vi "elab pictures 3d.vi"(8 "error in":errorcluster, 11 "path file in":path) -> (0 "error out":errorcluster)   [LabVIEW 2023]
uses:
  listbox/Selection Global Method.ctl
  <vilib>/Utility/file.llb/Read Delimited Spreadsheet (I64).vi
  queue/Front Panel Message Queue.lvlib
panel:
  in  "Z Slice":i16
  out "all rows 2":i32[][][](array[numeric])
  out "all rows":i32[][][](array[numeric])
  in  "List Selected":T1(array[cluster])
  out "List Selected v":string[](array[string])
  out "List File":i32(listbox)
  in  "load":bool
  in  "Stop":bool
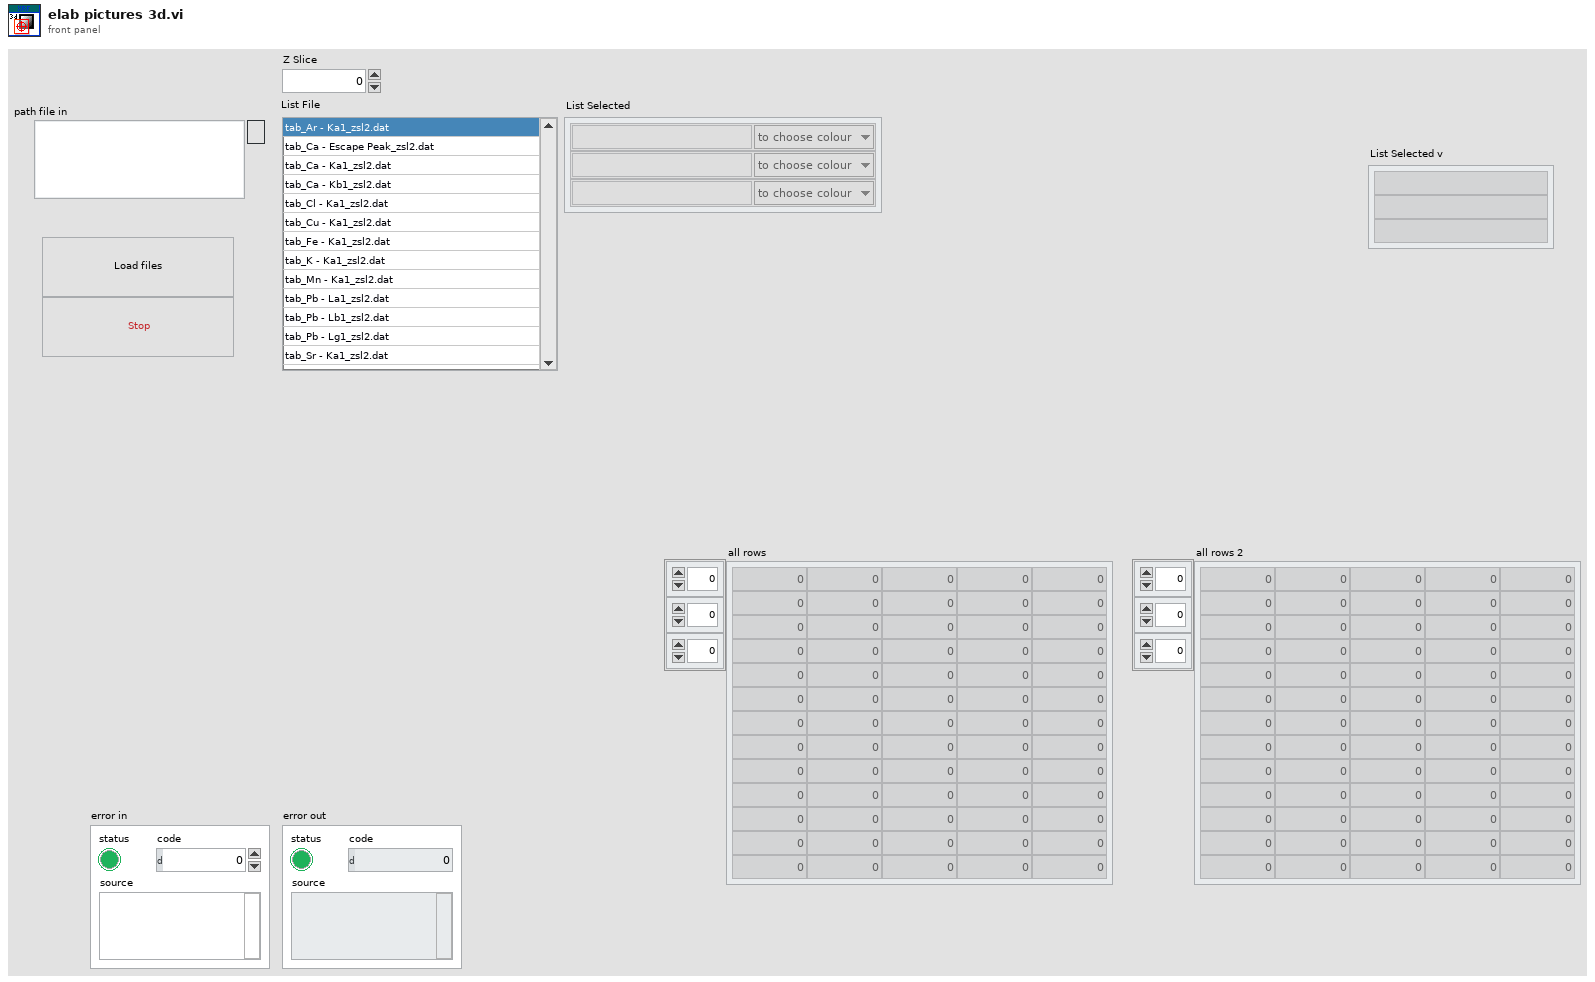
[diagram p1: front panel]
types:
  T1 = cluster{"Table":string, "color":enum16{"to choose colour", "red", "green", "blue"}}[]
  T2 = typedef "Front Panel Message Queue.lvlib/2d3d Message Queues.ctl" = cluster{"Main":refnum<queue>, "2d":refnum<queue>, "3d":refnum<queue>}
  T3 = typedef "Selection Global Method.ctl" = enum16{"Read Selection", "Force Selection", "Mouse Down Event", "Select All", "Select None", "Invert Selection", "Read Selection and Tags"}
  T4 = cluster{"Red name":string, "Green name":string, "Blu name":string}
  T5 = cluster{"Table":string, "color":enum16{"to choose colour", "red", "green", "blue"}}
  T6 = enum16{"to choose colour", "red", "green", "blue"}
  T7 = typedef "LVPoint32TypeDef.ctl" = cluster{"Horizontal":i32, "Vertical":i32}
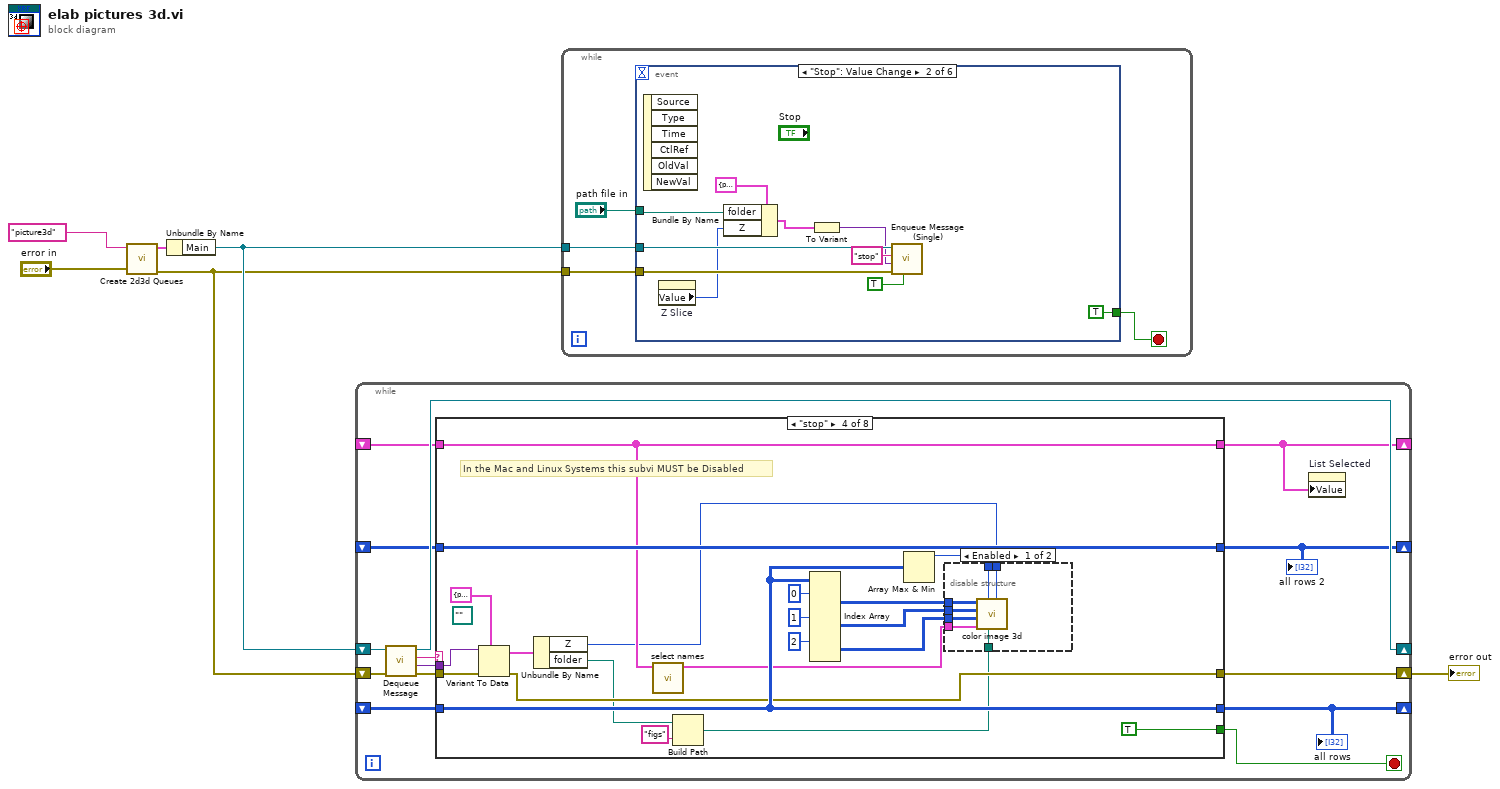
[diagram p0: block diagram]
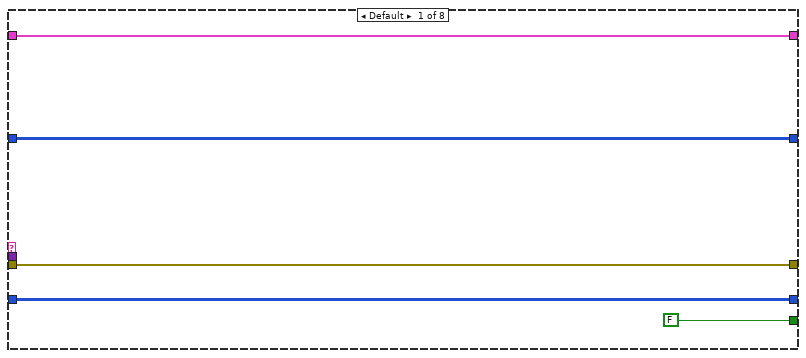
[diagram p2: hidden frame]
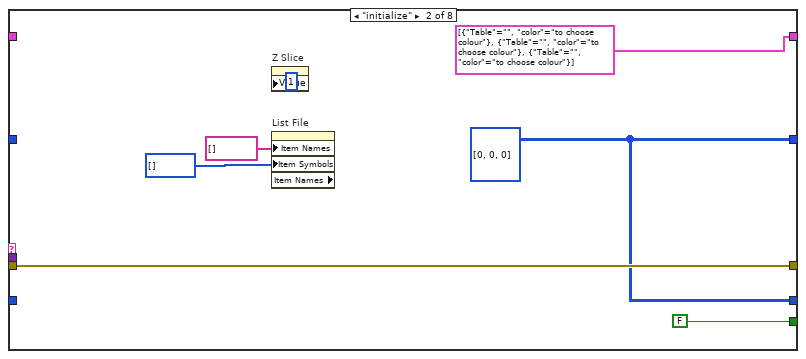
[diagram p3: hidden frame]
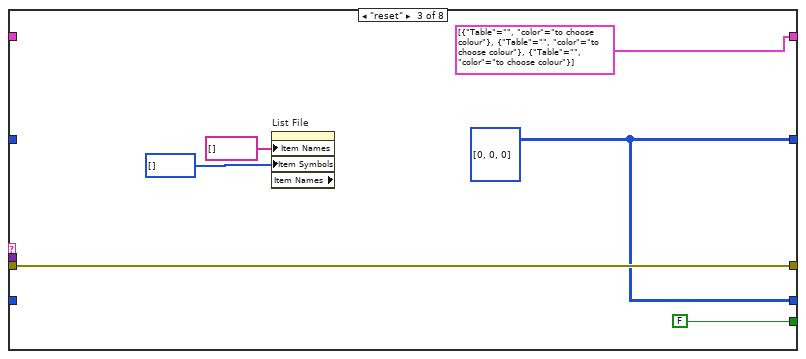
[diagram p4: hidden frame]
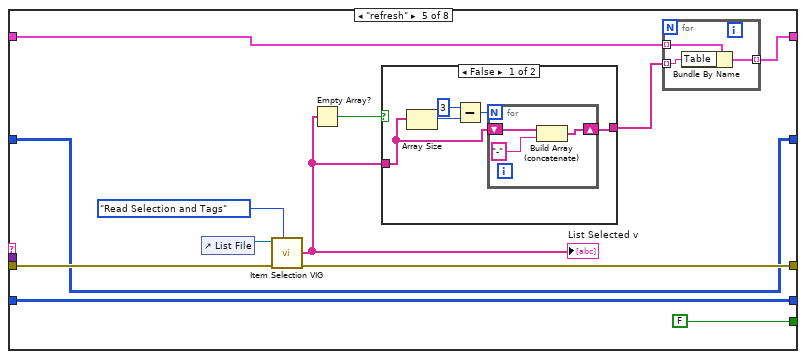
[diagram p6: hidden frame]
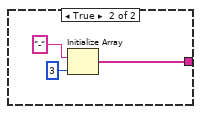
[diagram p7: hidden frame]
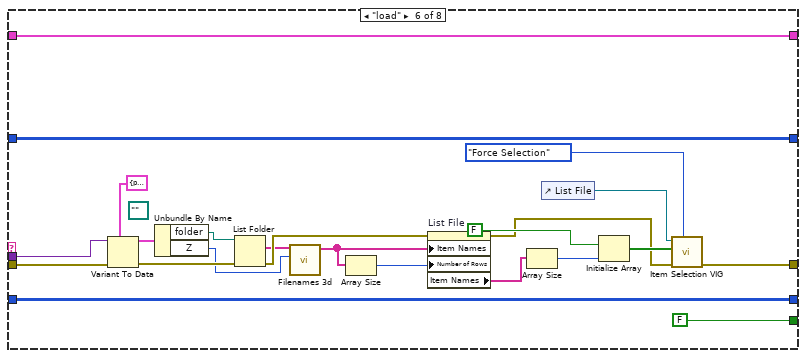
[diagram p8: hidden frame]
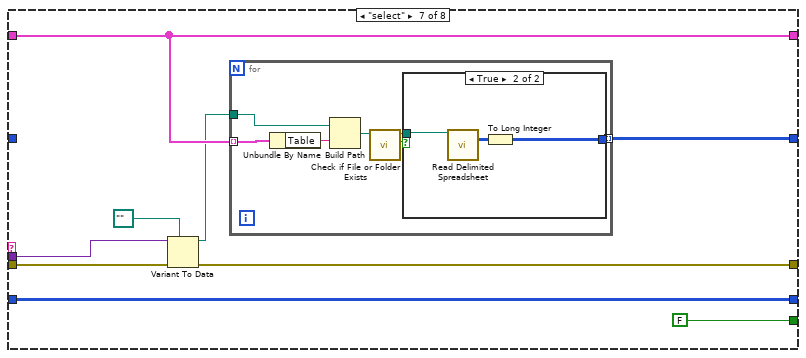
[diagram p9: hidden frame]
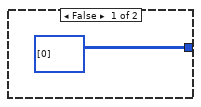
[diagram p10: hidden frame]
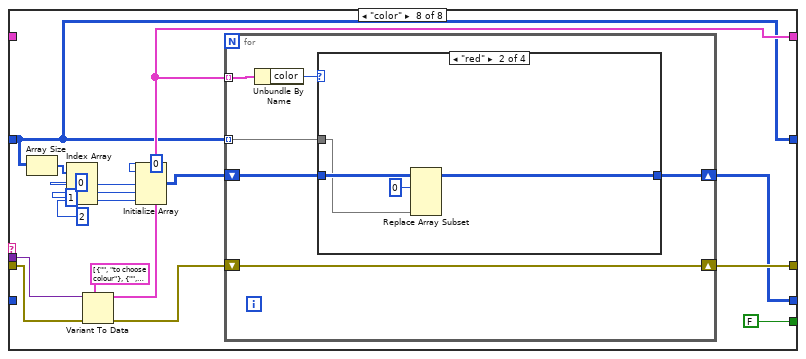
[diagram p11: hidden frame]
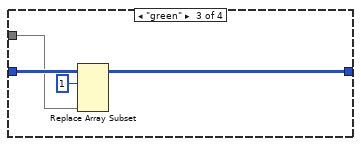
[diagram p13: hidden frame]
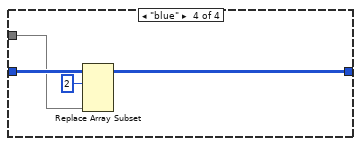
[diagram p14: hidden frame]
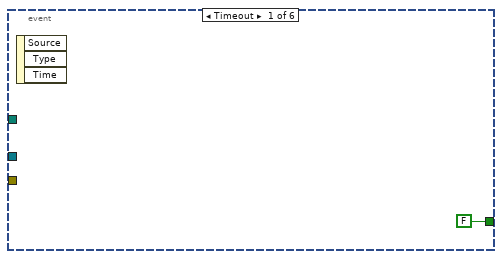
[diagram p15: hidden frame]
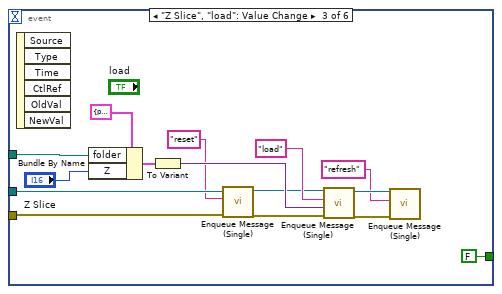
[diagram p16: hidden frame]
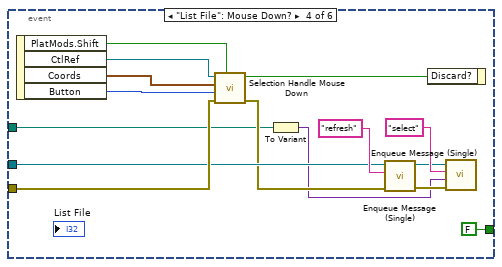
[diagram p17: hidden frame]
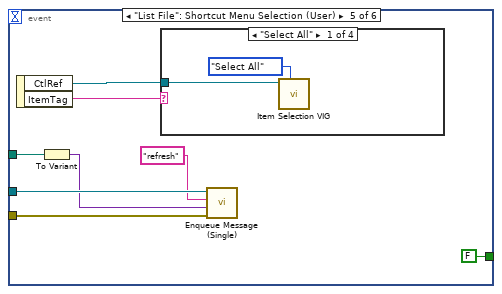
[diagram p18: hidden frame]
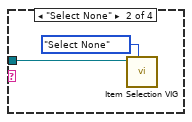
[diagram p19: hidden frame]
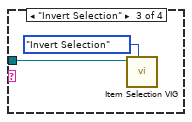
[diagram p20: hidden frame]
diagram:
  n1 = call "Create 2d3d Queues.vi"("error in (no error)"="error in", "name"="picture3d") -> ("error out"=w2:errorcluster, "Message Queues"=w4:T2)  [unwired: 8 in]
  n2 = Unbundle By Name(w4) -> ("Main"=w3:refnum<queue>)
  n3 = while {
    shift-right: [w13] -> _
    shift-left: w3 -> [w20]
    shift-right: [w17] -> w1
    shift-left: w2 -> [w19]
    shift-right: [w11] -> _
    shift-left: _ -> [w12]
    shift-right: [w10] -> _
    shift-left: _ -> [w9]
    shift-right: [w8] -> _
    shift-left: _ -> [w7]
    stop <- w15 stop-if-true
    n4 = call "Dequeue Message.vi"("error in (no error)"=w19, "Message Queue"=w20) -> ("error out"=w16:errorcluster, "Message Data"=w14:variant, "Message"=w18:string, "dup Message Queue"=w13:refnum<queue>)  [unwired: 5 in, 1 out]
    n5 = case shown="\"stop\"" w18 {
      tunnel: [w25 w29 w35 w45 w75 w102 w120 w152] -> w17
      tunnel: w16 -> [w25 w29 w35 w47 w74 w114 w123 w150]
      tunnel: [FALSE FALSE FALSE TRUE FALSE FALSE FALSE FALSE] -> w15
      tunnel: w14 -> [_ _ _ w46 _ w113 w121 w148]
      tunnel: w12 -> [w23 _ _ w49 w73 w101 w119 _]
      tunnel: [w23 T1 [{"Table"="", "color"=enum."to choose colour"}, {"Table"="", "color"=enum."to choose colour"}, {"Table"="", "color"=enum."to choose colour"}] ("List Selected") T1 [{"Table"="", "color"=enum."to choose colour"}, {"Table"="", "color"=enum."to choose colour"}, {"Table"="", "color"=enum."to choose colour"}] ("List Selected") w49 w72 w101 w119 w146] -> w11
      tunnel: [w22 w27 w33 w58 w68 w100 w117 w144] -> w10
      tunnel: w9 -> [w22 _ _ w58 w68 w100 _ w144]
      tunnel: [w21 w27 w33 w50 w67 w99 w116 w151] -> w8
      tunnel: w7 -> [w21 _ _ w50 w67 w99 w116 _]
      frame Default {
      }
      frame "initialize" {
        w27 = i32[][][] [[[0]], [[0]], [[0]]] ("all rows")
        n6 = property on="Z Slice" class="DigNum (strict)"("Value"=i16 1 ("Z")) -> ()  [unwired: 2 in, 2 out]
        n7 = property on="List File" class="LstBox (strict)" props=["Item Names", "Item Symbols", "Item Names"]("Item Names"=string[] [], "Item Symbols"=i32[] []) -> ()  [unwired: 2 in, 3 out]
      }
      frame "reset" {
        w33 = i32[][][] [[[0]], [[0]], [[0]]] ("all rows")
        n8 = property on="List File" class="LstBox (strict)" props=["Item Names", "Item Symbols", "Item Names"]("Item Names"=string[] [], "Item Symbols"=i32[] []) -> ()  [unwired: 2 in, 3 out]
      }
      frame "stop" {
        (unwired) path ""
        # "In the Mac and Linux Systems this subvi MUST be Disabled"
        n9 = Variant To Data(error in=w47, type=cluster{"folder":path, "Z":i16} {"folder"=path "", "Z"=0}, Variant=w46) -> (data=w41:cluster{"folder":path, "Z":i16}, error out=w45:errorcluster)
        n10 = Unbundle By Name(w41) -> ("Z"=w39:i16, "folder"=w40:path)
        n11 = call "select names.vi"("List Selected"=w49) -> ("Names"=w48:T4)  [unwired: 10 in]
        n12 = Build Path(base path=w40, name or relative path="figs") -> (appended path=w43:path)
        n13 = Index Array(array=w50, index (dim 0) #1=0 ("index (page)"), index (dim 0) #2=1 ("index (page)"), index (dim 0) #3=2 ("index (page)")) -> (element #1=w54:i32[][], element #2=w55:i32[][], element #3=w56:i32[][])  [unwired: 6 in]
        n14 = Array Max & Min(array=w50) -> (max value=w57:i32)  [unwired: 3 out]
        n15 = disable-structure shown="Enabled" {
          disable-tunnel: w57 -> [w66 _]
          disable-tunnel: w56 -> [w65 _]
          disable-tunnel: w55 -> [w64 _]
          disable-tunnel: w54 -> [w63 _]
          disable-tunnel: w48 -> [w62 _]
          disable-tunnel: w43 -> [w61 _]
          disable-tunnel: w39 -> [w60 _]
          frame Enabled {
            n16 = call "color image 3d.vi"("Z Slice"=w60, "path to JPEG file"=w61, "Max"=w66, "Names"=w62, "ROI-Blue"=w65, "ROI-Green"=w64, "ROI-Red"=w63) -> ()  [unwired: 5 in]
          }
          frame Disabled {
          }
        }
      }
      frame "refresh" {
        n17 = control-ref of="List File"() -> (w76:refnum<vi>)
        n18 = call "Item Selection VIG.vi"("Method (Read Selection)"=Selection_Global_Method."Read Selection and Tags", "error in (no error)"=w74, "Listbox or Tree"=w76) -> ("error out"=w75:errorcluster, "Tags"=w69:string[])  [unwired: 6 in, 1 out]
        "List Selected v" <- w69
        n19 = Empty Array?(array=w69) -> (empty?=w71:bool)
        n20 = case shown="False" w71 {
          tunnel: [w80 w87] -> w70
          tunnel: w69 -> [w79 _]
          frame False {
            n21 = Array Size(array=w79) -> (size(s)=w82:i32)
            n22 = Subtract(x=3, y=w82) -> (x-y=w83:i32)
            n23 = for {
              N: w83 -> [_]
              shift-right: [w84] -> w80
              shift-left: w79 -> [w86]
              n24 = Build Array (concatenate)(w86, "-") -> (w84:string[])
            }
          }
          frame True {
            n25 = Initialize Array("-", 3 ("dimension size")) -> (w87:string[])
          }
        }
        n26 = for {
          tunnel: w70 -> [w91] mode=indexing
          tunnel: w73 -> [w92] mode=indexing
          tunnel: [w90] -> w72 mode=indexing
          n27 = Bundle By Name(cluster=w92, "Table"=w91) -> (w90:T5)
        }
      }
      frame "load" {
        (unwired) path ""
        n28 = Variant To Data(error in=w114, type=cluster{"folder":path, "Z":i16} {"folder"=path "", "Z"=0}, Variant=w113) -> (data=w97:cluster{"folder":path, "Z":i16}, error out=w112:errorcluster)
        n29 = Unbundle By Name(w97) -> ("folder"=w96:path, "Z"=w93:i16)
        n30 = List Folder(path=w96, error in=w112) -> (filenames=w95:string[], error out=w111:errorcluster)  [unwired: 2 in, 2 out]
        n31 = call "Filenames 3d.vi"("Z Slice"=w93, "Filenames In"=w95) -> ("Filenames Out"=w94:string[])  [unwired: 9 in]
        n32 = Array Size(array=w94) -> (size(s)=w110:i32)
        n33 = property on="List File" class="LstBox (strict)"(error in=w111, "Item Names"=w94, "Number of Rows"=w110) -> (error out=w103:errorcluster, "Item Names"=w104:string[])  [unwired: 1 in, 1 out]
        n34 = Array Size(array=w104) -> (size(s)=w109:i32)
        n35 = control-ref of="List File"() -> (w108:refnum<vi>)
        n36 = Initialize Array(FALSE, w109) -> (w107:bool[])
        n37 = call "Item Selection VIG.vi"("Method (Read Selection)"=Selection_Global_Method."Force Selection", "error in (no error)"=w103, "Selection"=w107, "Listbox or Tree"=w108) -> ("error out"=w102:errorcluster)  [unwired: 5 in, 2 out]
      }
      frame "select" {
        n38 = Variant To Data(error in=w123, type=path "", Variant=w121) -> (data=w118:path, error out=w120:errorcluster)
        n39 = for {
          tunnel: w119 -> [w131] mode=indexing
          tunnel: w118 -> [w129]
          tunnel: [w125] -> w117 mode=indexing
          n40 = Unbundle By Name(w131) -> ("Table"=w130:string)
          n41 = Build Path(base path=w129, name or relative path=w130) -> (appended path=w128:path)
          n42 = call <vilib>:"Check if File or Folder Exists.vi"("path"=w128) -> ("file or folder exists?"=w127:bool, "dup path"=w126:path)  [unwired: 8 in, 1 out]
          n43 = case shown="True" w127 {
            tunnel: w126 -> [_ w135]
            tunnel: [i32[][] [[0]] ("all rows") w133] -> w125
            frame False {
            }
            frame True {
              n44 = call-poly <vilib>:"Read Delimited Spreadsheet.vi"("file path (dialog if empty)"=w135) -> ("all rows"=w134:i64[][])  [unwired: 9 in, 5 out]
              n45 = To Long Integer(number=w134) -> (32bit integer=w133:i32[][])
            }
          }
        }
      }
      frame "color" {
        n46 = Array Size(array=w144) -> (size(s)=w143:i32[])
        n47 = Index Array(array=w143, index #1=0 ("index"), index #2=1 ("index"), index #3=2 ("index")) -> (element #1=w139:i32, element #2=w138:i32, element #3=w137:i32)
        n48 = Variant To Data(error in=w150, type=T1 [{"Table"="", "color"=enum."to choose colour"}, {"Table"="", "color"=enum."to choose colour"}, {"Table"="", "color"=enum."to choose colour"}] ("List Selected"), Variant=w148) -> (data=w146:T1, error out=w149:errorcluster)
        n49 = Initialize Array(0, w139, w138, w137) -> (w136:i32[][][])
        n50 = for {
          tunnel: w146 -> [w158] mode=indexing
          tunnel: w144 -> [w156] mode=indexing
          shift-right: [w159] -> w152
          shift-left: w149 -> [w159]
          shift-right: [w154] -> w151
          shift-left: w136 -> [w155]
          n51 = Unbundle By Name(w158) -> ("color"=w157:T6)
          n52 = case shown="\"red\"" w157 {
            tunnel: w156 -> [_ w162 w166 w170]
            tunnel: w155 -> [w160 w164 w167 w171]
            tunnel: [w160 w161 w165 w169] -> w154
            frame "to choose colour", Default {
            }
            frame "red" {
              n53 = Replace Array Subset(array=w164, new element=w162, index (dim 0)=0 ("index (page)")) -> (w161:i32[][][])  [unwired: 2 in]
            }
            frame "green" {
              n54 = Replace Array Subset(array=w167, new element=w166, index (dim 0)=1 ("index (page)")) -> (w165:i32[][][])  [unwired: 2 in]
            }
            frame "blue" {
              n55 = Replace Array Subset(array=w171, new element=w170, index (dim 0)=2 ("index (page)")) -> (w169:i32[][][])  [unwired: 2 in]
            }
          }
        }
      }
    }
    "all rows" <- w8
    "all rows 2" <- w10
    n56 = property on="List Selected" class="Arr (strict)"("Value"=w11) -> ()  [unwired: 2 in, 2 out]
  }
  "error out" <- w1
  n57 = while {
    tunnel: w3 -> [w176]
    tunnel: w2 -> [w175]
    stop <- w174 stop-if-true
    n58 = event shown="[1] \"Stop\": Value Change" {
      selector: _ -> [_ _ _ _ _ _]
      dyn-events: _ -> [_ _ _ _ _ _]
      timeout: _ -> [_ _ _ _ _ _]
      tunnel: w176 -> [_ w186 w190 w209 w224 w236]
      tunnel: w175 -> [_ w185 w189 w211 w223 w237]
      tunnel: [FALSE TRUE FALSE FALSE FALSE FALSE] -> w174
      tunnel: "path file in" -> [_ w179 w194 w207 w221 _]
      event Timeout {
        n59 = event-data() -> ()  [unwired: 1 in, 3 out]
      }
      event "Stop": Value Change {
        n60 = event-data() -> ()  [unwired: 1 in, 6 out]
        n61 = property on="Z Slice" class="DigNum (strict)"() -> ("Value"=w180:i16)  [unwired: 2 in, 2 out]
        n62 = Bundle By Name(cluster=cluster{"folder":path, "Z":i16} {"folder"=path "", "Z"=0}, "folder"=w179, "Z"=w180) -> (w178:cluster{"folder":path, "Z":i16})
        n63 = To Variant(anything=w178) -> (Variant=w182:variant)
        n64 = call "Enqueue Message (Single).vi"("Priority Message? (F)"=TRUE, "error in (no error)"=w185, "Message Data"=w182, "Message"="stop", "Message Queue"=w186) -> ()  [unwired: 5 in, 2 out]
      }
      event "Z Slice", "load": Value Change {
        n65 = event-data() -> ()  [unwired: 1 in, 6 out]
        n66 = Bundle By Name(cluster=cluster{"folder":path, "Z":i16} {"folder"=path "", "Z"=0}, "folder"=w194, "Z"="Z Slice") -> (w196:cluster{"folder":path, "Z":i16})
        n67 = To Variant(anything=w196) -> (Variant=w200:variant)
        n68 = call "Enqueue Message (Single).vi"("error in (no error)"=w189, "Message"="reset", "Message Queue"=w190) -> ("error out"=w191:errorcluster, "dup Message Queue"=w192:refnum<queue>)  [unwired: 7 in]
        n69 = call "Enqueue Message (Single).vi"("error in (no error)"=w191, "Message Data"=w200, "Message"="load", "Message Queue"=w192) -> ("error out"=w199:errorcluster, "dup Message Queue"=w198:refnum<queue>)  [unwired: 6 in]
        n70 = call "Enqueue Message (Single).vi"("error in (no error)"=w199, "Message"="refresh", "Message Queue"=w198) -> ()  [unwired: 7 in, 2 out]
      }
      event "List File": Mouse Down? {
        n71 = event-data() -> ("PlatMods.Shift"=w213:bool, "CtlRef"=w214:refnum<vi>, "Coords"=w215:T7, "Button"=w216:u16)  [unwired: 1 in]
        n72 = call "Selection Handle Mouse Down.vi"("Shift?"=w213, "error in (no error)"=w211, "Mouse Button"=w216, "Mouse Coords"=w215, "Listbox or Tree"=w214) -> ("error out"=w208:errorcluster, "Discard?"=w212:bool)  [unwired: 5 in]
        n73 = To Variant(anything=w207) -> (Variant=w203:variant)
        n74 = call "Enqueue Message (Single).vi"("error in (no error)"=w208, "Message"="refresh", "Message Queue"=w209) -> ("error out"=w204:errorcluster, "dup Message Queue"=w205:refnum<queue>)  [unwired: 7 in]
        n75 = event-data("Discard?"=w212) -> ()  [unwired: 1 in, 1 out]
        n76 = call "Enqueue Message (Single).vi"("error in (no error)"=w204, "Message Data"=w203, "Message"="select", "Message Queue"=w205) -> ()  [unwired: 6 in, 2 out]
      }
      event "List File": Shortcut Menu Selection (User) {
        n77 = event-data() -> ("CtlRef"=w218:refnum<vi>, "ItemTag"=w219:string)  [unwired: 1 in]
        n78 = To Variant(anything=w221) -> (Variant=w220:variant)
        n79 = case shown="\"Select All\"" w219 {
          tunnel: w218 -> [w227 w229 w231 _]
          frame "Select All" {
            n80 = call "Item Selection VIG.vi"("Method (Read Selection)"=Selection_Global_Method."Select All", "Listbox or Tree"=w227) -> ()  [unwired: 7 in, 3 out]
          }
          frame "Select None" {
            n81 = call "Item Selection VIG.vi"("Method (Read Selection)"=Selection_Global_Method."Select None", "Listbox or Tree"=w229) -> ()  [unwired: 7 in, 3 out]
          }
          frame "Invert Selection" {
            n82 = call "Item Selection VIG.vi"("Method (Read Selection)"=Selection_Global_Method."Invert Selection", "Listbox or Tree"=w231) -> ()  [unwired: 7 in, 3 out]
          }
          frame Default {
          }
        }
        n83 = call "Enqueue Message (Single).vi"("error in (no error)"=w223, "Message Data"=w220, "Message"="refresh", "Message Queue"=w224) -> ()  [unwired: 6 in, 2 out]
      }
      event "List Selected": Value Change {
        n84 = event-data() -> ("NewVal"=w233:T1)  [unwired: 1 in, 5 out]
        n85 = To Variant(anything=w233) -> (Variant=w232:variant)
        n86 = call "Enqueue Message (Single).vi"("error in (no error)"=w237, "Message Data"=w232, "Message"="color", "Message Queue"=w236) -> ()  [unwired: 6 in, 2 out]
      }
    }
  }
